vi "_Replace Text in HTML.vi"(0 "HTML File Path":path, 5 "search string":string, 7 "replace string (\"\")":string, 11 "error in":errorcluster) -> (4 "HTML File Path out":path, 15 "error out":errorcluster)   [LabVIEW 2012]
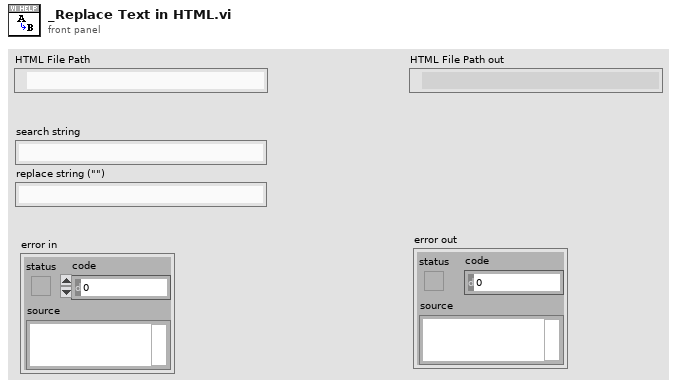
[diagram p1: front panel]
types:
  T1 = enum16{"open", "replace", "create", "open or create", "replace or create", "replace or create with confirmation"}
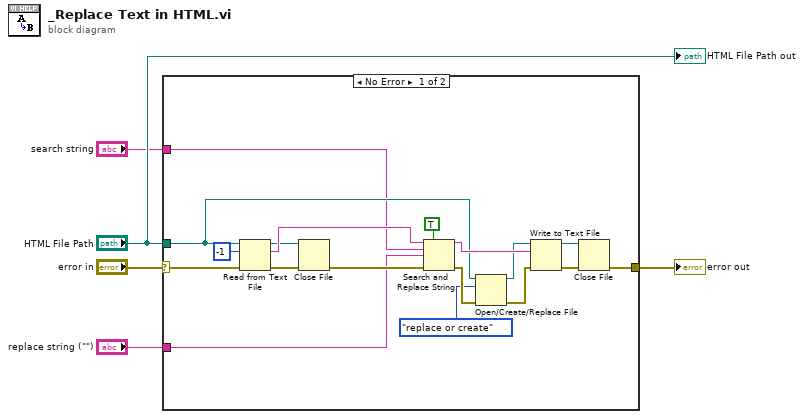
[diagram p0: block diagram]
diagram:
  n1 = case shown="No Error" "error in" {
    selector: "error in" -> [w6 w24]
    tunnel: "HTML File Path" -> [w12 _]
    tunnel: [w11 w24] -> w4
    tunnel: "search string" -> [w10 _]
    tunnel: "replace string (\"\")" -> [w9 _]
    frame No Error {
      n2 = Read from Text File(file (use dialog)=w12, count=-1, error in=w6) -> (refnum out=w17:refnum<file>, text=w20:string, error out=w18:errorcluster)  [unwired: 1 in, 1 out]
      n3 = Close File(refnum=w17, error in=w18) -> (error out=w16:errorcluster)  [unwired: 1 out]
      n4 = Search and Replace String(replace all?=TRUE ("replace all? (F)"), input string=w20, search string=w10, replace string=w9, error in=w16) -> (result string=w21:string, error out=w15:errorcluster)  [unwired: 3 in, 2 out]
      n5 = Open/Create/Replace File(file path (use dialog)=w12, error in=w15, operation (0:open)=T1."replace or create") -> (refnum out=w14:refnum<file>, error out=w13:errorcluster)  [unwired: 3 in, 1 out]
      n6 = Write to Text File(file (use dialog)=w14, text=w21, error in=w13) -> (refnum out=w23:refnum<file>, error out=w22:errorcluster)  [unwired: 1 in, 1 out]
      n7 = Close File(refnum=w23, error in=w22) -> (error out=w11:errorcluster)  [unwired: 1 out]
    }
    frame Error {
    }
  }
  "error out" <- w4
  "HTML File Path out" <- "HTML File Path"
